vi "Enqueue Message (Single).vi"(6 "Message prioritaire ? (F)":bool, 8 "error in (no error)":T1 caption="entrée d'erreur (pas d'erreur)", 9 "Données de message":variant, 10 "Message":string, 11 "File d'attente de messages":refnum<queue>) -> (0 "error out":T1 caption="sortie d'erreur", 3 "File d'attente de message dup.":refnum<queue>)   [LabVIEW 2020, in "Message Queue.lvlib"]
doc: "Pour un message normal, placer le message à la fin de la file d'attente. Pour un message prioritaire, l'ajouter au début de la file."
uses:
  Message Queue.lvlib
  Message Cluster.ctl
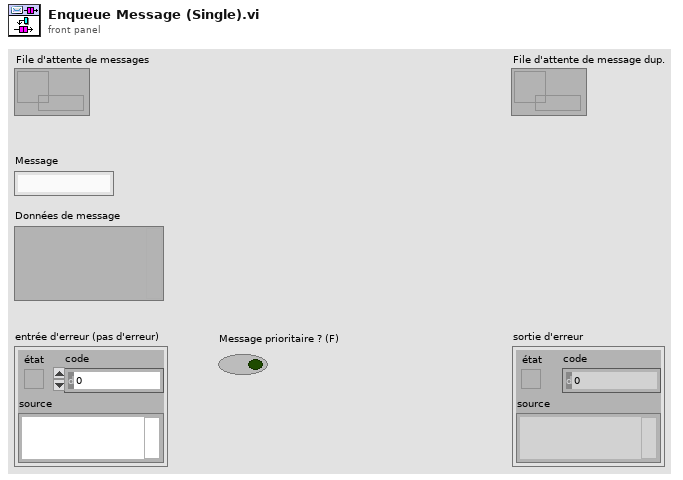
[diagram p1: front panel]
types:
  T1 = cluster{"état":bool, "code":i32, "source":string}
  T2 = typedef "Message Queue.lvlib/Message Cluster.ctl" = cluster{"Message":string, "Données de message":variant}
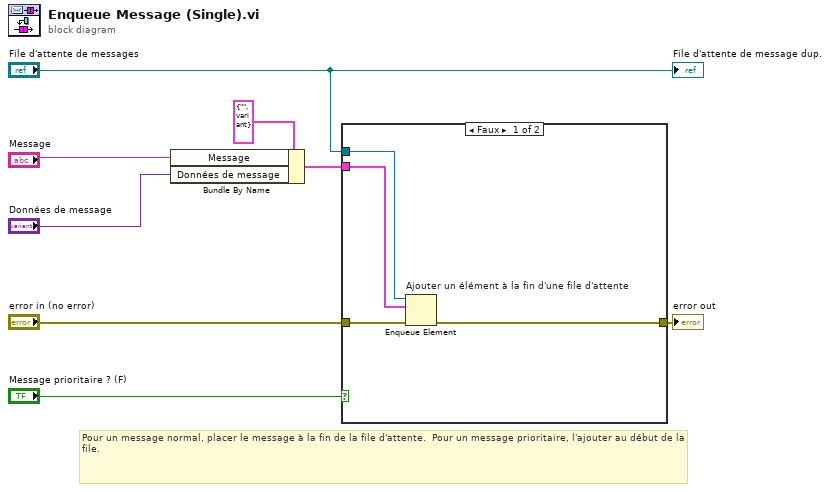
[diagram p0: block diagram]
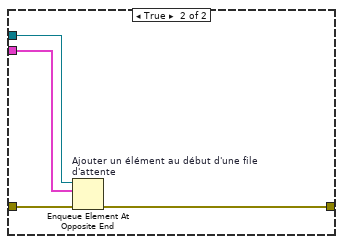
[diagram p2: hidden frame]
diagram:
  # "Pour un message normal, placer le message à la fin de la file d'attente.  Pour un message prioritaire, l'ajouter au début de la file."
  n1 = Bundle By Name(cluster=T2 {"Message"="", "Données de message"=variant} ("Message Cluster"), "Message"="Message", "Données de message"="Données de message") -> (w1:T2)
  n2 = case shown="Faux" "Message prioritaire ? (F)" {
    tunnel: "error in (no error)" -> [w12 w16]
    tunnel: [w11 w15] -> w3
    tunnel: "File d'attente de messages" -> [w10 w14]
    tunnel: w1 -> [w9 w13]
    frame False {
      n3 = Enqueue Element "Ajouter un élément à la fin d'une file d'attente"(queue=w10, element=w9, error in (no error)=w12) -> (error out=w11:errorcluster)  [unwired: 1 in, 2 out]
    }
    frame True {
      n4 = Enqueue Element At Opposite End "Ajouter un élément au début d'une file d'attente"(queue=w14, element=w13, error in (no error)=w16) -> (error out=w15:errorcluster)  [unwired: 1 in, 2 out]
    }
  }
  "error out" <- w3
  "File d'attente de message dup." <- "File d'attente de messages"
